vi "string_to_array.vi"(10 "program string":string) -> (2 "array":string[](array[string]))   [LabVIEW 2015]
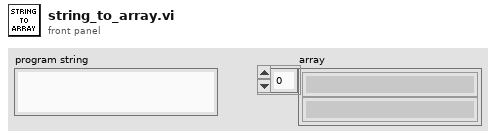
[diagram p1: front panel]
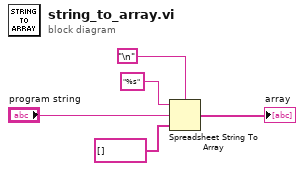
[diagram p0: block diagram]
diagram:
  n1 = Spreadsheet String To Array(delimiter (Tab)="\n", format string="%s", spreadsheet string="program string", array type (2D Dbl)=string[] []) -> (array=→"array":string[])
